vi "Open.vi"(0 "reference in":refnum<class "UDS.lvclass">, 5 "error in (no error)":errorcluster) -> (14 "reference out":refnum<class "UDS.lvclass">, 19 "error out":errorcluster)   [LabVIEW 2020, in "UDS.lvclass"]
uses:
  UDS.lvclass
  <vilib>/addons/Automotive Diagnostic Command Set/NI_Automotive Diagnostic Command Set.lvlib
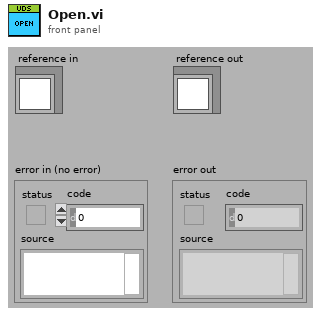
[diagram p1: front panel]
types:
  T1 = typedef "UDS.lvclass/ObjectAttributesRef.ctl" = refnum<data-value>
  T2 = typedef "UDS.lvclass/ObjectAttributes.ctl" = cluster{"MyAttribute":dbl, "UDSSetting":cluster{"InterfacName":string, "Baud Rate":u64, "FD Baud Rate":u64, "Transport Protocol":T3, "IO Mode":u32, "Max DLC":u16, "Transmit ID":u32, "Receive ID":u32, "Wait Time CF (STmin)":u32, "Fill Byte":u32}, "diag ref":T4}
  T3 = typedef "NI_Automotive Diagnostic Command Set.lvlib/Transport Protocol Selector.ctl" = enum16{"ISO TP - Normal Mode", "ISO TP - Mixed Mode", "VW TP 2.0", "Diagnostics on IP", "ISO TP LIN"}
  T4 = typedef "NI_Automotive Diagnostic Command Set.lvlib/Diag Reference.ctl" = cluster{"Diag CAN Handle":u32, "Transport Protocol":T3, "Receive Address Extension":u8, "Transmit Address Extension":u8, "Receive CAN Id":u32, "Transmit CAN Id":u32, "Log Frames ?":bool, "My TP Address":u8, "Other TP Address":u8, "T1":u16, "T2":u16, "T3":u16, "T4":u16, "Tx SN":u8, "Block Size":u8, "Rx SN":u8, "VW TP Initialized?":bool, "Tx block no":u8, "baud rate":u64, "Interface":string, "Channel Diag CAN Handle":u32, "UDP Connection ID":refnum<k16>, "TCP Connection ID":refnum<k5>, "Target IP Addr":u32, "Source Address":u16, "Target Address":u16, "Send Header NACK?":bool, "DLL Handle":u32, "NAD":u8, "Time Stamp read first":dbl, "Time Stamp read last":dbl, "Time Stamp write first":dbl, "Time Stamp write last":dbl, "Time Stamp write":dbl, "Time Stamp read":dbl, " I/O Mode":u32, "FD Baudrate":u64, "TX_DL":u16, "RX_DL":u16, "DoIP Protocol Version":T5, " Selected I/O Mode":u32, "TesterPresent Counter":u32, "TesterPresent Limit":u32, "TesterPresent Tick[ms]":i32, "TesterPresent RequireResponse?":bool, "TesterPresent Stored Ref?":bool, "TesterPresent Message":u8[], "TesterPresent Task Handle":i32, "TesterPresent Semaphore":T6, "Response Plausibility Check":u32, "Default Version?":bool, "Diagostic Globals":T7, "Session-based Properties?":bool}
  T5 = typedef "NI_Automotive Diagnostic Command Set.lvlib/DoIP Protocol Version.ctl" = u8
  T6 = typedef "Semaphore RefNum" = refnum<k1>
  T7 = typedef "NI_Automotive Diagnostic Command Set.lvlib/Diag Globals.ctl" = cluster{"Timeout FC (Bs)":u32, "Timeout CF (Cr)":u32, "Timeout Diag Command":u32, "Receive Block Size (BS)":u8, "Wait Time CF (STmin)":u8, "Max Waits (N_WFTmax)":u8, "Waits to Send (N_WAIT)":i32, "Time between Waits (TW)":u32, "Fill CAN Frames?":bool, "Fill Byte":u32, "Invalid Response as Error?":bool, "Max RspPending Count":u32, "VWTP Command Timeout":u32, "Transport Protocol":T3, "Diag CAN Handle":u32, "DLL Handle":u32, "Timeout RspPending":u32}
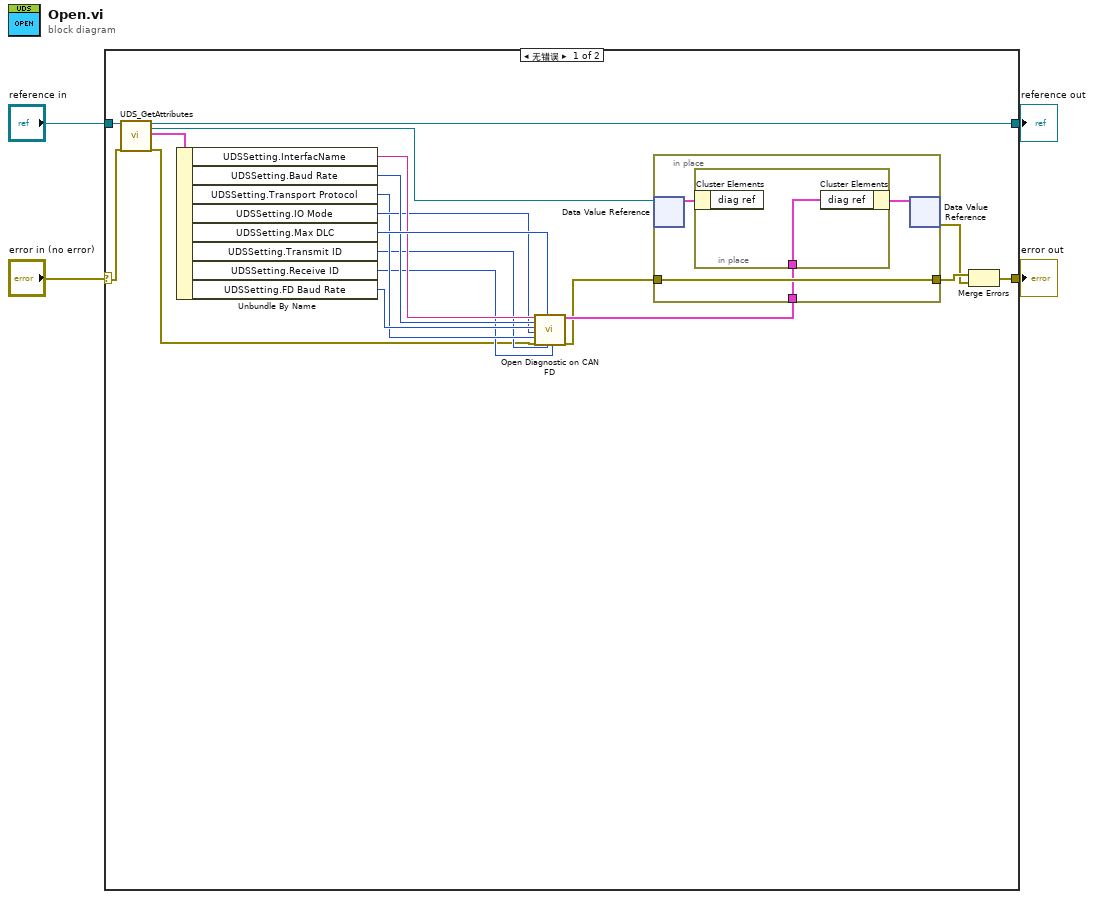
[diagram p0: block diagram]
diagram:
  n1 = case shown="无错误" "error in (no error)" {
    selector: "error in (no error)" -> [w20 w30]
    tunnel: [w23 w30] -> w3
    tunnel: [w21 w29] -> w1
    tunnel: "reference in" -> [w22 w29]
    frame No Error {
      n2 = call "UDS_GetAttributes.vi"("reference in"=w22, "error in (no error)"=w20) -> ("reference out"=w21:refnum<class "UDS.lvclass">, "attributes ref"=w16:T1, "attributes"=w19:T2, "error out"=w6:errorcluster)  [unwired: 14 in]
      n3 = Unbundle By Name(w19) -> ("UDSSetting.InterfacName"=w14:string, "UDSSetting.Baud Rate"=w13:u64, "UDSSetting.Transport Protocol"=w10:T3, "UDSSetting.IO Mode"=w11:u32, "UDSSetting.Max DLC"=w15:u16, "UDSSetting.Transmit ID"=w9:u32, "UDSSetting.Receive ID"=w8:u32, "UDSSetting.FD Baud Rate"=w12:u64)
      n4 = call <vilib>:"Open Diagnostic on CAN FD.vi"("CAN Interface"=w14, "Baud Rate"=w13, "FD Baud Rate"=w12, "IO Mode"=w11, "Transport Protocol"=w10, "error in (no error)"=w6, "Max DLC"=w15, "Transmit ID"=w9, "Receive ID"=w8) -> ("diag ref out"=w7:T4, "error out"=w5:errorcluster)  [unwired: 9 in]
      n5 = in-place {
        in-place-border: w5 -> [w25]
        in-place-border: [w25] -> w18
        in-place-border: w7 -> [w24]
        n6 = in-place-dvr #1(w16) -> (w26:T2)  [unwired: 1 out]
        n7 = in-place {
          in-place-border: w24 -> [w28]
          n8 = in-place-cluster #2(w26) -> ()  [unwired: 1 out]
          n9 = in-place-cluster #2("diag ref"=w28) -> (w27:T2)
        }
        n10 = in-place-dvr #1(w27) -> (w17:errorcluster)  [unwired: 1 out]
      }
      n11 = Merge Errors(w18, w17) -> (w23:errorcluster)
    }
    frame Error {
    }
  }
  "error out" <- w3
  "reference out" <- w1
